vi "libversion.vi"(8 "error in (no error)":errorcluster) -> (0 "error out":errorcluster, 1 "Minor":i32, 2 "Major":i32, 3 "Version String":string, 4 "Fix":i32)   [LabVIEW 2015]
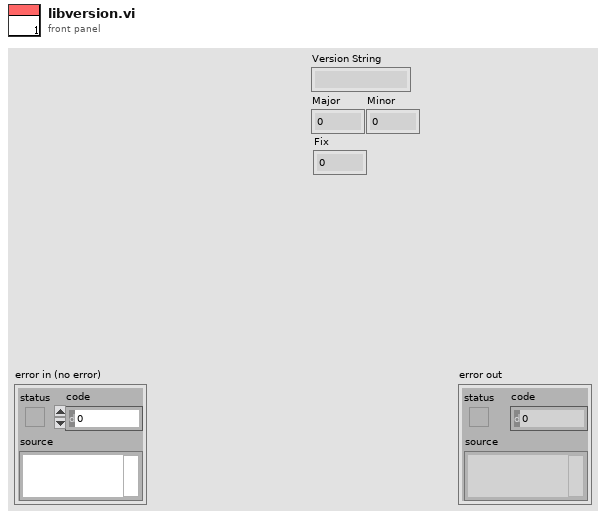
[diagram p1: front panel]
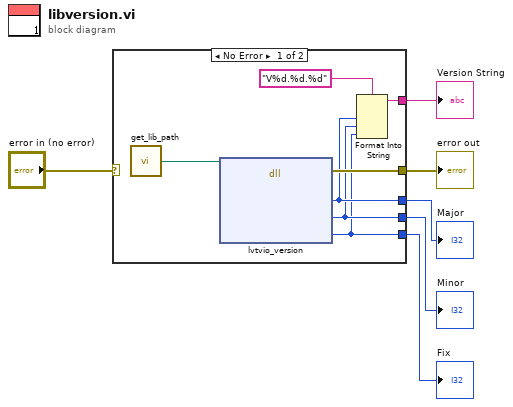
[diagram p0: block diagram]
diagram:
  n1 = case shown="No Error" "error in (no error)" {
    selector: "error in (no error)" -> [_ w14]
    tunnel: [w12 w14] -> w5
    tunnel: [w10 _] -> w4
    tunnel: [w9 _] -> w3
    tunnel: [w8 _] -> w2
    tunnel: [w7 _] -> w1
    frame No Error {
      n2 = call "get_lib_path.vi"() -> ("Path"=w13:path)
      n3 = dll-call lib="S:/thingiverselv/lib/liblvtvio.dll" fn="lvtvio_version"(path in=w13) -> (error out=w12:errorcluster, "maj"=w9:i32, "min"=w8:i32, "version"=w7:i32)  [unwired: 6 in, 1 out]
      n4 = Format Into String(format string="V%d.%d.%d" ("result"), w9, w8, w7) -> (resulting string=w10:string)  [unwired: 2 in, 1 out]
    }
    frame Error {
    }
  }
  "error out" <- w5
  "Version String" <- w4
  "Minor" <- w2
  "Fix" <- w1
  "Major" <- w3
